vi "Timer Count with Error Handling.vi"(6 "Reset":bool, 8 "error in (no error)":errorcluster) -> (0 "error out":errorcluster, 2 "Elapsed Time (ms)":u32)   [LabVIEW 2018, in "Utilities.lvlib"]
uses:
  Utilities.lvlib
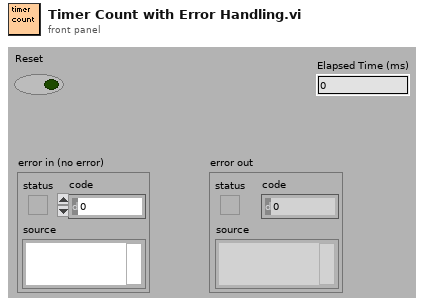
[diagram p1: front panel]
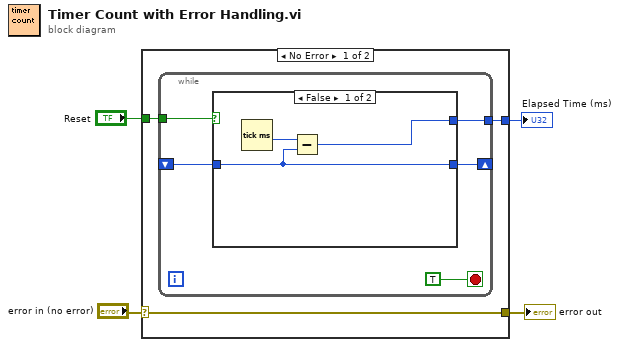
[diagram p0: block diagram]
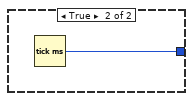
[diagram p2: hidden frame]
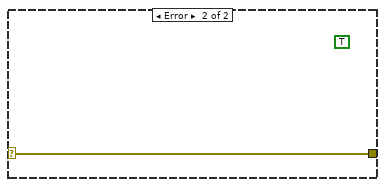
[diagram p3: hidden frame]
diagram:
  n1 = case shown="No Error" "error in (no error)" {
    selector: "error in (no error)" -> [w7 w17]
    tunnel: [w7 w17] -> w3
    tunnel: "Reset" -> [w6 _]
    tunnel: [w5 _] -> w1
    frame No Error {
      n2 = while {
        shift-right: [w11] -> _
        shift-left: _ -> [w9]
        tunnel: w6 -> [w10]
        tunnel: [w8] -> w5
        stop <- TRUE stop-if-true
        n3 = case shown="False" w10 {
          tunnel: [w14 w16] -> w11
          tunnel: w9 -> [w14 _]
          tunnel: [w13 _] -> w8
          frame False {
            n4 = Tick Count (ms)() -> (millisecond timer value=w15:u32)
            n5 = Subtract(x=w15, y=w14) -> (x-y=w13:u32)
          }
          frame True {
            n6 = Tick Count (ms)() -> (millisecond timer value=w16:u32)
          }
        }
      }
    }
    frame Error {
      (unwired) TRUE
    }
  }
  "error out" <- w3
  "Elapsed Time (ms)" <- w1
